vi "test-diff-drive-kinematics.vi"(8 "error in (no error)":errorcluster) -> (0 "error out":errorcluster, 3 "All Passed":bool)   [LabVIEW 2019]
uses:
  <vilib>/Rock Robotics/SystemInterfaces/NetworkCommunication/NetComm_UsageReport_report.vi
  <vilib>/Rock Robotics/WPI/ThirdParty/JAS_Junk/TrajLib/Util_LibraryGlobals.vi
  <vilib>/Rock Robotics/WPI/ThirdParty/JAS_Junk/TrajLib/Trajectory_Library.lvlib
panel:
  out "Passed Test 5":bool
  out "Passed Test 4":bool
  out "Passed Test 3":bool
  out "Passed Test 2":bool
  out "Passed Test 1":bool
  out "Passed Test 0":bool
  # "Diff Drive Kinematic Test"
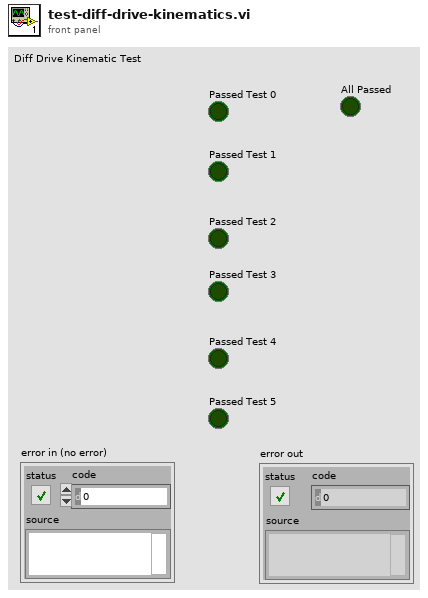
[diagram p1: front panel]
types:
  T1 = typedef "Trajectory_Library.lvlib/CHASSIS_SPEEDS.ctl" = cluster{"vX":dbl, "vY":dbl, "vOmega":dbl}
  T2 = typedef "Trajectory_Library.lvlib/DIFF_DRIVE_KINEMATICS.ctl" = cluster{"TrackWidth_Meters":dbl}
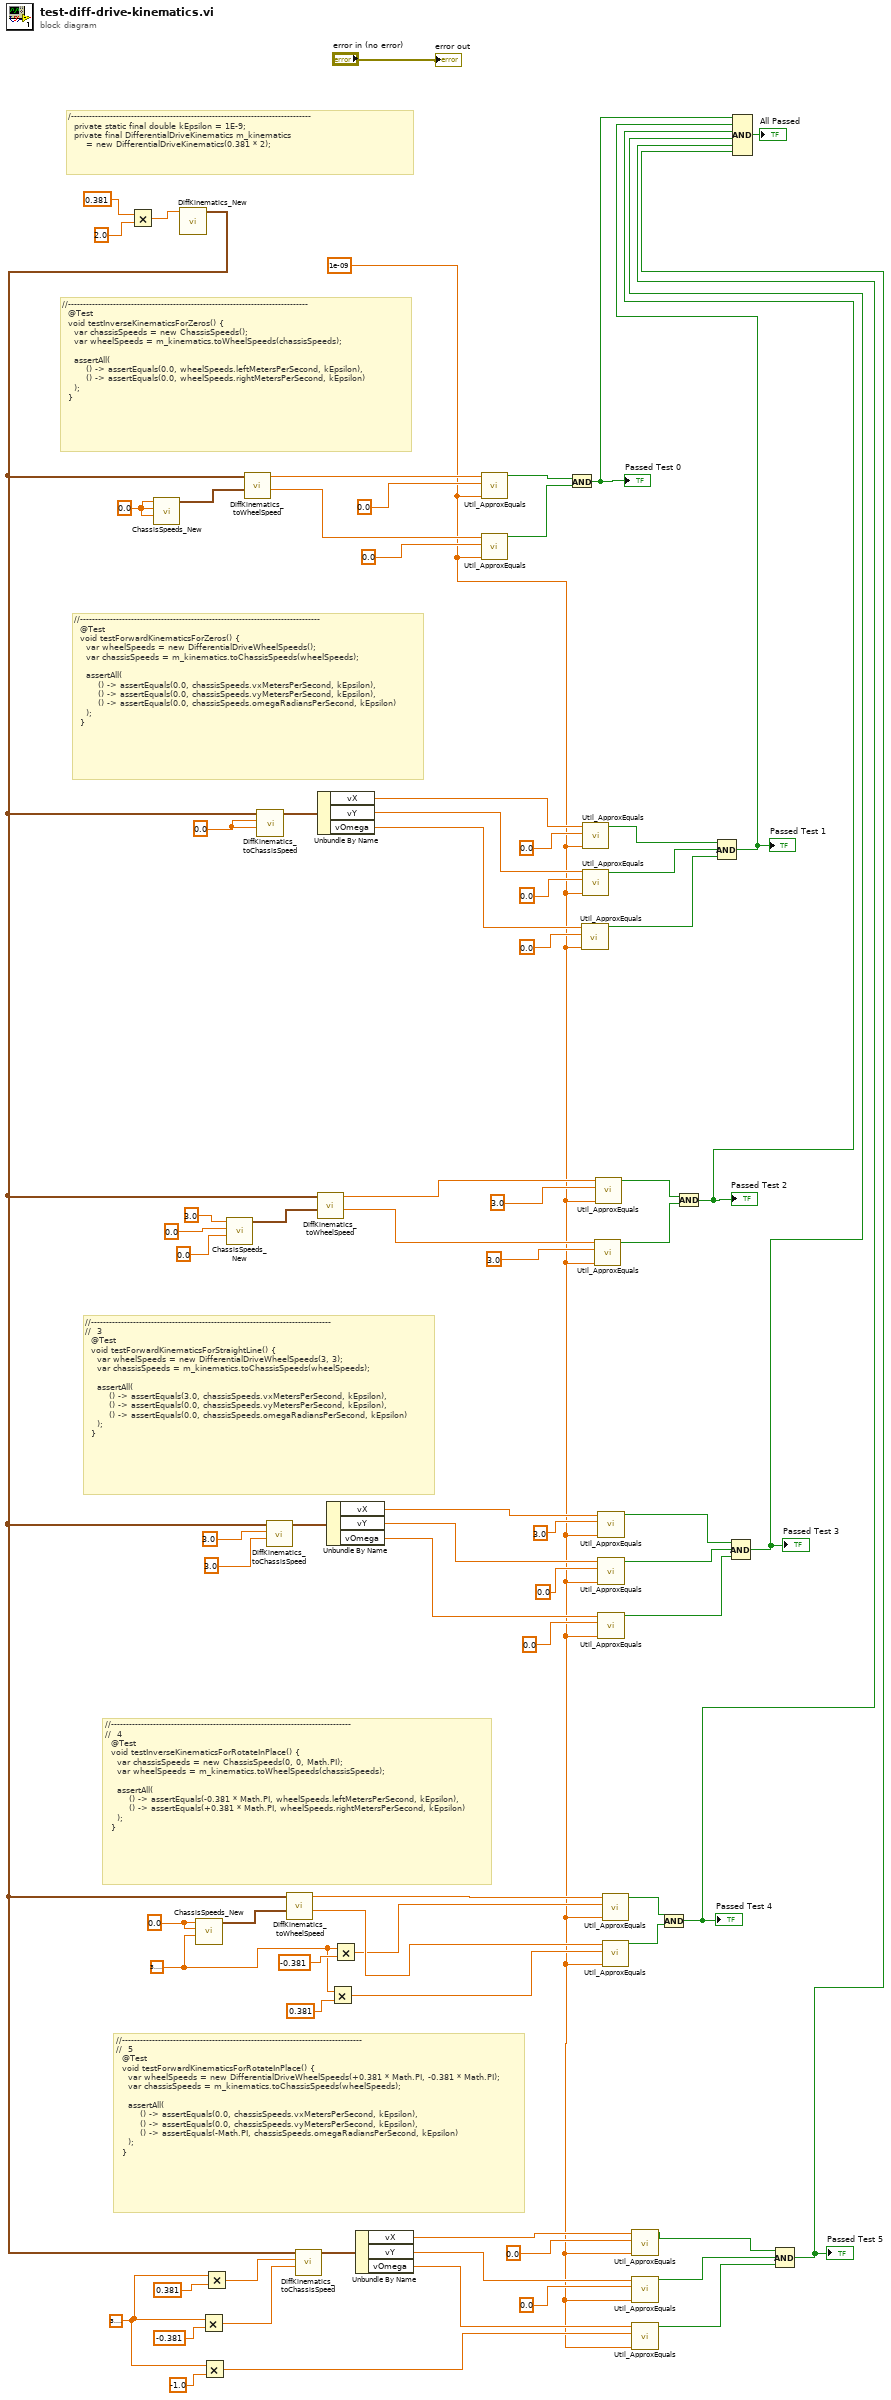
[diagram p0: block diagram]
diagram:
  w2 = 1e-09 ("y")
  w55 = 3.141592653589793
  w63 = 3.141592653589793
  w67 = 0.0 ("vX")
  w76 = 0.0 ("LeftVelocity")
  w78 = 0.0 ("vX")
  # "//--------------------------------------------------------------------------------\n//  5\n  @Test\n  void testForwardKinematicsForRotateInPlace() {\n    var wheelSpeeds = new DifferentialDriveWheelSpeeds(+0.381 * Math.PI, -0.381 * Math.PI);\n    var chassisSpeeds = m_kinematics.toChassisSpeeds(wheelSpeeds);\n\n    assertAll(\n        () -> assertEquals(0.0, chassisSpeeds.vxMetersPerSecond, kEpsilon),\n        () -> assertEquals(0.0, chassisSpeeds.vyMetersPerSecond, kEpsilon),\n        () -> assertEquals(-Math.PI, chassisSpeeds.omegaRadiansPerSecond, kEpsilon)\n    );\n  }"
  # "//--------------------------------------------------------------------------------\n//  4\n  @Test\n  void testInverseKinematicsForRotateInPlace() {\n    var chassisSpeeds = new ChassisSpeeds(0, 0, Math.PI);\n    var wheelSpeeds = m_kinematics.toWheelSpeeds(chassisSpeeds);\n\n    assertAll(\n        () -> assertEquals(-0.381 * Math.PI, wheelSpeeds.leftMetersPerSecond, kEpsilon),\n        () -> assertEquals(+0.381 * Math.PI, wheelSpeeds.rightMetersPerSecond, kEpsilon)\n    );\n  }"
  # "//--------------------------------------------------------------------------------\n//  3\n  @Test\n  void testForwardKinematicsForStraightLine() {\n    var wheelSpeeds = new DifferentialDriveWheelSpeeds(3, 3);\n    var chassisSpeeds = m_kinematics.toChassisSpeeds(wheelSpeeds);\n\n    assertAll(\n        () -> assertEquals(3.0, chassisSpeeds.vxMetersPerSecond, kEpsilon),\n        () -> assertEquals(0.0, chassisSpeeds.vyMetersPerSecond, kEpsilon),\n        () -> assertEquals(0.0, chassisSpeeds.omegaRadiansPerSecond, kEpsilon)\n    );\n  }"
  # "//--------------------------------------------------------------------------------\n  @Test\n  void testForwardKinematicsForZeros() {\n    var wheelSpeeds = new DifferentialDriveWheelSpeeds();\n    var chassisSpeeds = m_kinematics.toChassisSpeeds(wheelSpeeds);\n\n    assertAll(\n        () -> assertEquals(0.0, chassisSpeeds.vxMetersPerSecond, kEpsilon),\n        () -> assertEquals(0.0, chassisSpeeds.vyMetersPerSecond, kEpsilon),\n        () -> assertEquals(0.0, chassisSpeeds.omegaRadiansPerSecond, kEpsilon)\n    );\n  }"
  # "/--------------------------------------------------------------------------------\n  private static final double kEpsilon = 1E-9;\n  private final DifferentialDriveKinematics m_kinematics\n      = new DifferentialDriveKinematics(0.381 * 2);"
  # "//--------------------------------------------------------------------------------\n  @Test\n  void testInverseKinematicsForZeros() {\n    var chassisSpeeds = new ChassisSpeeds();\n    var wheelSpeeds = m_kinematics.toWheelSpeeds(chassisSpeeds);\n\n    assertAll(\n        () -> assertEquals(0.0, wheelSpeeds.leftMetersPerSecond, kEpsilon),\n        () -> assertEquals(0.0, wheelSpeeds.rightMetersPerSecond, kEpsilon)\n    );\n  }"
  n1 = Multiply(x=0.381, y=2.0) -> (x*y=w79:dbl)
  n2 = call <vilib>:"ChassisSpeeds_New.vi"("vAngular"=w78, "vY"=w78, "vX"=w78) -> ("CHASSIS"=w77:T1)  [unwired: 8 in]
  n3 = call <vilib>:"DiffKinematics_New.vi"("TrackWidth_Meters"=w79) -> ("DIFF_DRIVE_KINEMATICS"=w61:T2)  [unwired: 10 in]
  n4 = call <vilib>:"ChassisSpeeds_New.vi"("vAngular"=w63, "vY"=w67, "vX"=w67) -> ("CHASSIS"=w66:T1)  [unwired: 8 in]
  n5 = Multiply(x=w55, y=-0.381) -> (x*y=w57:dbl)
  n6 = Multiply(x=w55, y=-1.0) -> (x*y=w14:dbl)
  n7 = Multiply(x=w55, y=0.381) -> (x*y=w58:dbl)
  n8 = call <vilib>:"ChassisSpeeds_New.vi"("vAngular"=0.0, "vY"=0.0, "vX"=3.0) -> ("CHASSIS"=w74:T1)  [unwired: 8 in]
  n9 = call <vilib>:"DiffKinematics_toWheelSpeed.vi"("CHASSIS Speed"=w77, "DIFF_DRIVE_KINEMATICS"=w61) -> ("RightVelocity"=w46:dbl, "LeftVelocity"=w47:dbl)  [unwired: 8 in]
  n10 = call <vilib>:"DiffKinematics_toChassisSpeed.vi"("RightVelocity"=w76, "LeftVelocity"=w76, "inDIFF_DRIVE_KINEMATICS"=w61) -> ("CHASSIS Speed"=w75:T1)  [unwired: 8 in]
  n11 = call <vilib>:"DiffKinematics_toChassisSpeed.vi"("RightVelocity"=3.0, "LeftVelocity"=3.0, "inDIFF_DRIVE_KINEMATICS"=w61) -> ("CHASSIS Speed"=w69:T1)  [unwired: 8 in]
  n12 = call <vilib>:"DiffKinematics_toWheelSpeed.vi"("CHASSIS Speed"=w66, "DIFF_DRIVE_KINEMATICS"=w61) -> ("RightVelocity"=w6:dbl, "LeftVelocity"=w5:dbl)  [unwired: 8 in]
  n13 = call <vilib>:"DiffKinematics_toChassisSpeed.vi"("RightVelocity"=w57, "LeftVelocity"=w58, "inDIFF_DRIVE_KINEMATICS"=w61) -> ("CHASSIS Speed"=w62:T1)  [unwired: 8 in]
  n14 = Unbundle By Name(w75) -> ("vX"=w41:dbl, "vY"=w40:dbl, "vOmega"=w39:dbl)
  n15 = call <vilib>:"DiffKinematics_toWheelSpeed.vi"("CHASSIS Speed"=w74, "DIFF_DRIVE_KINEMATICS"=w61) -> ("RightVelocity"=w30:dbl, "LeftVelocity"=w32:dbl)  [unwired: 8 in]
  n16 = Unbundle By Name(w69) -> ("vX"=w23:dbl, "vY"=w22:dbl, "vOmega"=w21:dbl)
  n17 = Multiply(x=w63, y=0.381) -> (x*y=w3:dbl)
  n18 = Multiply(x=w63, y=-0.381) -> (x*y=w4:dbl)
  n19 = Unbundle By Name(w62) -> ("vX"=w17:dbl, "vY"=w16:dbl, "vOmega"=w15:dbl)
  n20 = call <vilib>:"Util_ApproxEquals.vi"("Tolerance"=w2, "Value 2"=0.0 ("y"), "Value 1"=w47) -> ("ApproxEquals"=w43:bool)  [unwired: 8 in]
  n21 = call <vilib>:"Util_ApproxEquals.vi"("Tolerance"=w2, "Value 2"=0.0 ("y"), "Value 1"=w46) -> ("ApproxEquals"=w42:bool)  [unwired: 8 in]
  n22 = And(x=w43, y=w42) -> (x .and. y?=w54:bool)
  "Passed Test 0" <- w54
  n23 = call <vilib>:"Util_ApproxEquals.vi"("Tolerance"=w2, "Value 2"=0.0 ("y"), "Value 1"=w39) -> ("ApproxEquals"=w33:bool)  [unwired: 8 in]
  n24 = call <vilib>:"Util_ApproxEquals.vi"("Tolerance"=w2, "Value 2"=0.0 ("y"), "Value 1"=w41) -> ("ApproxEquals"=w35:bool)  [unwired: 8 in]
  n25 = call <vilib>:"Util_ApproxEquals.vi"("Tolerance"=w2, "Value 2"=0.0 ("y"), "Value 1"=w40) -> ("ApproxEquals"=w34:bool)  [unwired: 8 in]
  n26 = call <vilib>:"Util_ApproxEquals.vi"("Tolerance"=w2, "Value 2"=3.0 ("y"), "Value 1"=w30) -> ("ApproxEquals"=w27:bool)  [unwired: 8 in]
  n27 = call <vilib>:"Util_ApproxEquals.vi"("Tolerance"=w2, "Value 2"=3.0 ("y"), "Value 1"=w32) -> ("ApproxEquals"=w28:bool)  [unwired: 8 in]
  n28 = call <vilib>:"Util_ApproxEquals.vi"("Tolerance"=w2, "Value 2"=3.0 ("y"), "Value 1"=w23) -> ("ApproxEquals"=w26:bool)  [unwired: 8 in]
  n29 = call <vilib>:"Util_ApproxEquals.vi"("Tolerance"=w2, "Value 2"=0.0 ("y"), "Value 1"=w22) -> ("ApproxEquals"=w25:bool)  [unwired: 8 in]
  n30 = call <vilib>:"Util_ApproxEquals.vi"("Tolerance"=w2, "Value 2"=0.0 ("y"), "Value 1"=w21) -> ("ApproxEquals"=w24:bool)  [unwired: 8 in]
  n31 = call <vilib>:"Util_ApproxEquals.vi"("Tolerance"=w2, "Value 2"=w4, "Value 1"=w5) -> ("ApproxEquals"=w8:bool)  [unwired: 8 in]
  n32 = call <vilib>:"Util_ApproxEquals.vi"("Tolerance"=w2, "Value 2"=w3, "Value 1"=w6) -> ("ApproxEquals"=w7:bool)  [unwired: 8 in]
  n33 = call <vilib>:"Util_ApproxEquals.vi"("Tolerance"=w2, "Value 2"=0.0 ("y"), "Value 1"=w17) -> ("ApproxEquals"=w11:bool)  [unwired: 8 in]
  n34 = call <vilib>:"Util_ApproxEquals.vi"("Tolerance"=w2, "Value 2"=0.0 ("y"), "Value 1"=w16) -> ("ApproxEquals"=w10:bool)  [unwired: 8 in]
  n35 = call <vilib>:"Util_ApproxEquals.vi"("Tolerance"=w2, "Value 2"=w14, "Value 1"=w15) -> ("ApproxEquals"=w9:bool)  [unwired: 8 in]
  n36 = Compound Arithmetic op=AND(w8, w7) -> (w50:bool)
  "Passed Test 4" <- w50
  n37 = Compound Arithmetic op=AND(w28, w27) -> (w52:bool)
  "Passed Test 2" <- w52
  n38 = Compound Arithmetic op=AND(w35, w34, w33) -> (w53:bool)
  "Passed Test 1" <- w53
  n39 = Compound Arithmetic op=AND(w26, w25, w24) -> (w51:bool)
  "Passed Test 3" <- w51
  n40 = Compound Arithmetic op=AND(w11, w10, w9) -> (w49:bool)
  "Passed Test 5" <- w49
  n41 = Compound Arithmetic op=AND(w54, w53, w52, w51, w50, w49) -> (→"All Passed":bool)
  "error out" <- "error in (no error)"
